vi "Broadcast State (Data Map).vi"(8 "error in":errorcluster, 10 "Data Table":map{string, dbl}(c390)) -> (0 "error out":errorcluster)   [LabVIEW 2024, in "FlexiFlowInterfaceCH2.lvlib"]
doc: "Broadcasts the state in a data map.\n_____\nCreated using DQMH Event Scripter 7.0.1.1316."
uses:
  FlexiFlowInterfaceCH2.lvlib
  Broadcast State (Data Map) Argument--cluster.ctl
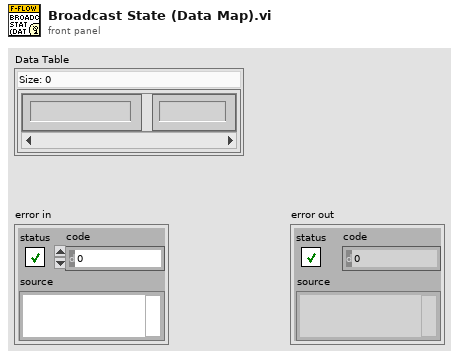
[diagram p1: front panel]
types:
  T1 = typedef "FlexiFlowInterfaceCH2.lvlib/Broadcast State (Data Map) Argument--cluster.ctl" = cluster{"Data Table":map{string, dbl}}
  T2 = typedef "FlexiFlowInterfaceCH2.lvlib/Broadcast Events--cluster.ctl" = cluster{"Module Did Init":refnum<user-event>, "Status Updated":refnum<user-event>, "Error Reported":refnum<user-event>, "Module Did Stop":refnum<user-event>, "Update Module Execution Status":refnum<user-event>, "Broadcast Device States":refnum<user-event>, "Broadcast State (Data Map)":refnum<user-event>}
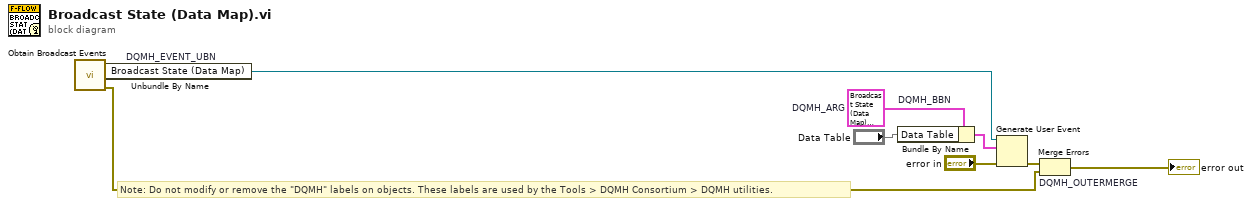
[diagram p0: block diagram]
diagram:
  w4 = T1 {"Data Table"={}}  # DQMH_ARG
  # "Note: Do not modify or remove the \"DQMH\" labels on objects. These labels are used by the Tools > DQMH Consortium > DQMH utilities."
  n1 = call "Obtain Broadcast Events.vi"() -> ("error out"=w2:errorcluster, "FlexiFlowInterfaceCH2 Broadcast Events"=w1:T2)  [unwired: 10 in]
  n2 = Unbundle By Name "DQMH_EVENT_UBN"(w1) -> ("Broadcast State (Data Map)"=w6:refnum<user-event>)
  n3 = Bundle By Name "DQMH_BBN"(cluster=w4, "Data Table"="Data Table") -> (w7:T1)
  n4 = Generate User Event(user event=w6, event data cluster=w7, error in="error in") -> (error out=w5:errorcluster)  [unwired: 1 in, 1 out]
  n5 = Merge Errors "DQMH_OUTERMERGE"(w5, w2) -> (→"error out":errorcluster)
